vi "Enqueue Message (Array).vi"(6 "Priority Message? Array":bool[](array[boolean]) caption="优先消息？数组", 8 "error in (no error)":errorcluster caption="错误输入（无错误）", 9 "Message Data Array":variant[](array[variant]) caption="消息数据数组", 10 "Message Array":string[](array[string]) caption="消息数组", 11 "Message Queue":refnum<queue> caption="消息队列") -> (0 "error out":errorcluster caption="错误输出", 3 "dup Message Queue":refnum<queue> caption="消息队列副本")   [LabVIEW 2015, in "Message Queue.lvlib"]
doc: "对于标准消息，将消息加入队列。对于优先消息，将消息加入队列的头部。"
uses:
  Message Queue.lvlib
  Message Cluster.ctl
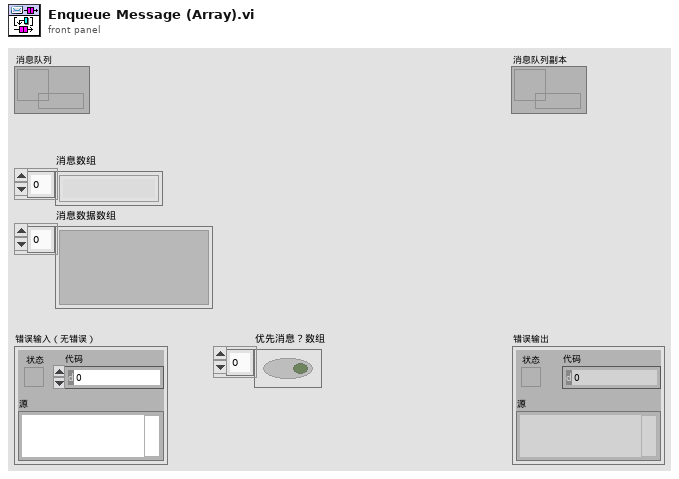
[diagram p1: front panel]
types:
  T1 = typedef "Message Queue.lvlib/Message Cluster.ctl" = cluster{"Message":string, "Message Data":variant}
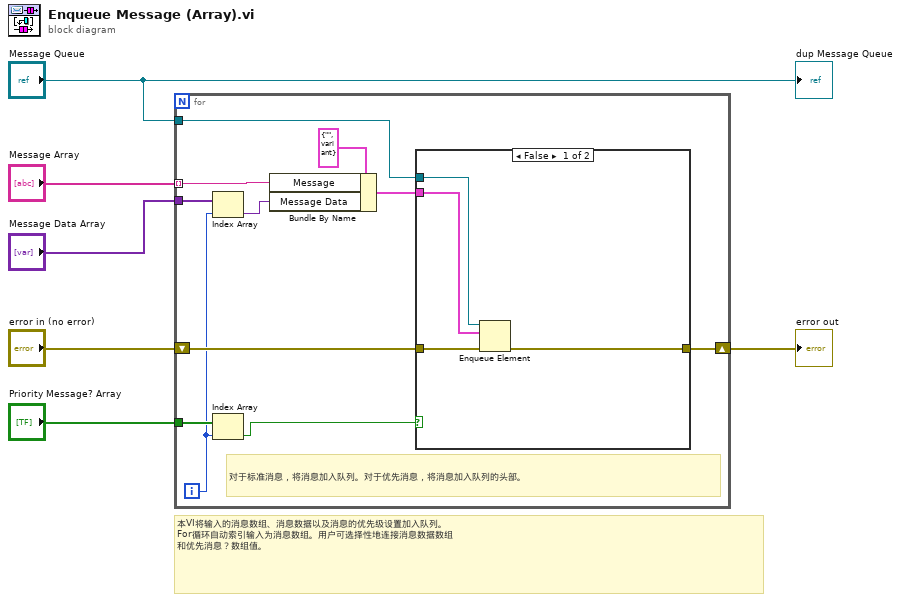
[diagram p0: block diagram]
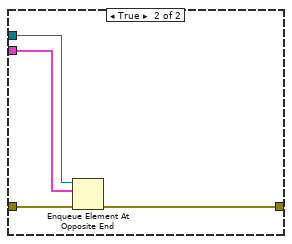
[diagram p2: hidden frame]
diagram:
  # "本VI将输入的消息数组、消息数据以及消息的优先级设置加入队列。\nFor循环自动索引输入为消息数组。用户可选择性地连接消息数据数组\n和优先消息？数组值。"
  n1 = for {
    tunnel: "Message Queue" -> [w14]
    tunnel: "Message Array" -> [w12] mode=indexing
    tunnel: "Message Data Array" -> [w11]
    tunnel: "Priority Message? Array" -> [w9]
    shift-right: [w15] -> w5
    shift-left: "error in (no error)" -> [w16]
    i -> [w7]
    # "对于标准消息，将消息加入队列。对于优先消息，将消息加入队列的头部。"
    n2 = Index Array(array=w11, index=w7) -> (element=w10:variant)
    n3 = Index Array(array=w9, index=w7) -> (element=w8:bool)
    n4 = Bundle By Name(cluster=T1 {"Message"="", "Message Data"=variant} ("Message Cluster"), "Message"=w12, "Message Data"=w10) -> (w13:T1)
    n5 = case shown="False" w8 {
      tunnel: w16 -> [w21 w25]
      tunnel: [w20 w24] -> w15
      tunnel: w14 -> [w19 w23]
      tunnel: w13 -> [w18 w22]
      frame False {
        n6 = Enqueue Element(queue=w19, element=w18, error in (no error)=w21) -> (error out=w20:errorcluster)  [unwired: 1 in, 2 out]
      }
      frame True {
        n7 = Enqueue Element At Opposite End(queue=w23, element=w22, error in (no error)=w25) -> (error out=w24:errorcluster)  [unwired: 1 in, 2 out]
      }
    }
  }
  "error out" <- w5
  "dup Message Queue" <- "Message Queue"
